vi "make_axes_grid_planes.vi"(10 "Scene Object In":refnum<vi>) -> (2 "Scene Object Out":refnum<vi>)   [LabVIEW 2020, in "3DPC_SurfacePlot.xctl"]
uses:
  <vilib>/Native 3D Graph/xcontrol/3DPC_SurfacePlot.xctl
  <vilib>/Native 3D Graph/typedefs/prop_axes_merged_array_etc.ctl
  <vilib>/Native 3D Graph/typedefs/prop_axes_merged_array.ctl
  <vilib>/Native 3D Graph/typedefs/range_cluster.ctl
  <vilib>/Native 3D Graph/typedefs/min_max.ctl
  <vilib>/Native 3D Graph/typedefs/prop_axes_grid.ctl
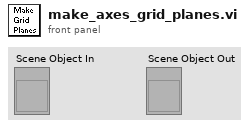
[diagram p1: front panel]
types:
  T1 = typedef "3DPC_SurfacePlot.xctl/prop_axes_merged_array_etc.ctl" = cluster{"X Merged Array":T2, "Y Merged Array":T2, "Z Merged Array":T2, "Range Min/Max":T3}
  T2 = typedef "3DPC_SurfacePlot.xctl/prop_axes_merged_array.ctl" = cluster{"Show Tick":bool, "Show Line":bool, "Interval":sgl, "Name":string}[]
  T3 = typedef "3DPC_SurfacePlot.xctl/range_cluster.ctl" = cluster{"X":T4, "Y":T4, "Z":T4, "Amplitude":T4}
  T4 = typedef "3DPC_SurfacePlot.xctl/min_max.ctl" = cluster{"Min":sgl, "Max":sgl}
  T5 = typedef "3DPC_SurfacePlot.xctl/prop_axes_grid.ctl" = cluster{"Grid Visible":cluster{"Draw X-grid":bool, "Draw Y-grid":bool, "Draw Z-grid":bool}, "Grid Color":cluster{"Color X":u32, "Color Y":u32, "Color Z":u32}}
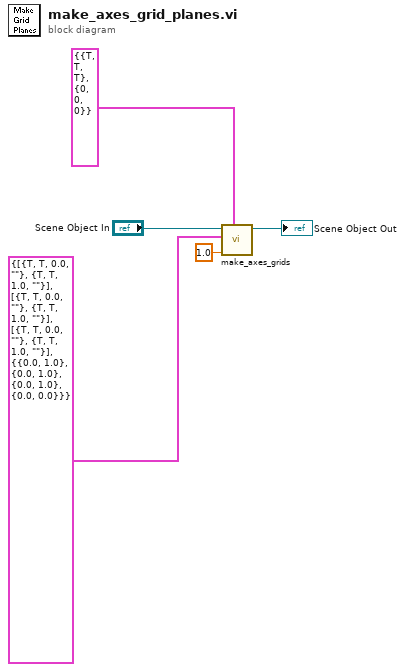
[diagram p0: block diagram]
diagram:
  n1 = call <vilib>:"make_axes_grids.vi"("Grid  Properties"=T5 {"Grid Visible"={"Draw X-grid"=TRUE, "Draw Y-grid"=TRUE, "Draw Z-grid"=TRUE}, "Grid Color"={"Color X"=0, "Color Y"=0, "Color Z"=0}}, "length"=sgl 1.0, "Axis output cluster"=T1 {"X Merged Array"=[{"Show Tick"=TRUE, "Show Line"=TRUE, "Interval"=0.0, "Name"=""}, {"Show Tick"=TRUE, "Show Line"=TRUE, "Interval"=1.0, "Name"=""}], "Y Merged Array"=[{"Show Tick"=TRUE, "Show Line"=TRUE, "Interval"=0.0, "Name"=""}, {"Show Tick"=TRUE, "Show Line"=TRUE, "Interval"=1.0, "Name"=""}], "Z Merged Array"=[{"Show Tick"=TRUE, "Show Line"=TRUE, "Interval"=0.0, "Name"=""}, {"Show Tick"=TRUE, "Show Line"=TRUE, "Interval"=1.0, "Name"=""}], "Range Min/Max"={"X"={"Min"=0.0, "Max"=1.0}, "Y"={"Min"=0.0, "Max"=1.0}, "Z"={"Min"=0.0, "Max"=1.0}, "Amplitude"={"Min"=0.0, "Max"=0.0}}}, "Scene Object In"="Scene Object In") -> ("Scene Object Out"=→"Scene Object Out":refnum<vi>)  [unwired: 1 in, 6 out]
